vi "Analysis_ELV_From_CVS.vi"() -> ()   [LabVIEW 2018]
uses:
  <vilib>/Utility/file.llb/Read Delimited Spreadsheet (DBL).vi
  <vilib>/imath/engines/lvmath2/RunTimeEngine/RangeToken/NIMS_Range.vi
  <instcachedir>/0/NIMS_Range_846134F467D14A349F7C6CCEF459CDB2.lvgen/NIMS_Range_846134F467D14A349F7C6CCEF459CDB2_000.vi
  <vilib>/imathl/engines/lvmath/Functions/Error Handling/Create Error.vi
  <vilib>/imath/engines/lvmath2/RunTimeEngine/BuiltInFunctions/length/NIMS_length(GV).vi
  <instcachedir>/0/NIMS_length(GV)_08A3D13377FD4E4B96F5795FBF3698FA.lvgen/NIMS_length(GV)_08A3D13377FD4E4B96F5795FBF3698FA_000.vi
  <vilib>/imath/engines/lvmath2/RunTimeEngine/RangeToken/NIMS_Range_R2 - Integer.vi
  <instcachedir>/0/NIMS_Range_R2 - Integer_E35B921DECF84AADB7325A02D418BFCC.lvgen/NIMS_Range_R2 - Integer_E35B921DECF84AADB7325A02D418BFCC_000.vi
  <vilib>/imath/engines/lvmath2/RunTimeEngine/CommandStatement/MC_CommandStatement_break.vi
  <vilib>/imath/engines/lvmath2/RunTimeEngine/IndexRead/NIMS V(S).vi
  <instcachedir>/0/NIMS V(S)_0488751826AF41519A22953C041130DC.lvgen/NIMS V(S)_0488751826AF41519A22953C041130DC_000.vi
  <vilib>/imath/engines/lvmath2/RunTimeEngine/BuiltInFunctions/rem/NIMS_rem_no checks.vi
  <instcachedir>/0/NIMS_rem_no checks_268F985FDA964107BCCF66D5C0ADFD07.lvgen/NIMS_rem_no checks_268F985FDA964107BCCF66D5C0ADFD07_000.vi
  <vilib>/imath/engines/lvmath2/RunTimeEngine/VariableToken/NIMS_VariableToken_CondDefinedDefinedByReplace.vi
  <instcachedir>/0/NIMS_VariableToken_CondDefinedDefinedByReplace_D162CFFC24174562A9FEA619A91E1A56.lvgen/NIMS_VariableToken_CondDefinedDefinedByReplace_D162CFFC24174562A9FEA619A91E1A56_002.vi
  <vilib>/imath/engines/lvmath2/RunTimeEngine/IndexReplace/NIMS V(S)=S.vi
  <instcachedir>/0/NIMS V(S)=S_420DA4522869420292A92FA3CC108C4E.lvgen/NIMS V(S)=S_420DA4522869420292A92FA3CC108C4E_000.vi
  <vilib>/imath/engines/lvmath2/RunTimeEngine/VariableToken/NIMS_VariableToken_CondDefined.vi
  <instcachedir>/0/NIMS_VariableToken_CondDefined_BADDB804EBCA4B86883699DABD34B224.lvgen/NIMS_VariableToken_CondDefined_BADDB804EBCA4B86883699DABD34B224_003.vi
  <vilib>/imath/engines/lvmath2/RunTimeEngine/BuiltInFunctions/interpolate1d/NIMS_interpolate1d(RV,RV,RV,Str).vi
  <vilib>/imath/engines/lvmath2/RunTimeEngine/ErrorHandling/NIMS_Create Error From Enums.vi
  <vilib>/imath/engines/lvmath/Functions/Error Handling/MergeErrorsWrapper.vi
  <vilib>/imath/engines/lvmath2/RunTimeEngine/NodeEndStatement/NIMS_NodeEndStatement_Output.vi
  <instcachedir>/0/NIMS_NodeEndStatement_Output_53EC0D466D134D7ABD903AC30B43404B.lvgen/NIMS_NodeEndStatement_Output_53EC0D466D134D7ABD903AC30B43404B_001.vi
  <instcachedir>/0/NIMS_NodeEndStatement_Output_53EC0D466D134D7ABD903AC30B43404B.lvgen/NIMS_NodeEndStatement_Output_53EC0D466D134D7ABD903AC30B43404B_005.vi
  <vilib>/imath/engines/lvmath2/RunTimeEngine/ErrorHandling/NIMS_Finalize Error.vi
panel:
  out "out2":dbl=0.071713257355
  out "out1":dbl=0.0297284806645
  in  "Tab Control":T1(tab)=enum."Confirming tn equation by comparing curves"
  out "Before Normalization":cluster{"all rows":dbl[], "all rows":dbl[]}(graph)
  out "After Normalization":cluster{"all rows":dbl[], "all rows":dbl[]}(graph)
  out "Emax":dbl=3.25
  out "tmax":dbl=0.2957
  out "E0":dbl=0.006655 format="%_10g"
  in  "Ed":dbl=0.006655
  in  "b":dbl=0.3
  in  "a":dbl=0.16
  in  "Num Cycles":dbl=5.0
  in  "HR":dbl=90.0
  in  "dt":dbl=0.0001
  in  "t0":dbl
  out "XY Graph":cluster{"tnvec":dbl[], "Ev":dbl[]}[](graph)
  out "min value":dbl
  in  "After normalization":path=path "C:/Users/suraj/Documents/Academic/Thesis - Physiological Control/From Ethan/Model1_EKF_12stateCVS/From_CVS_ELV_Norm.txt"
  in  "Original from Jeff":path=path "C:/Users/suraj/Documents/Academic/Thesis - Physiological Control/From Ethan/Model1_EKF_12stateCVS/From_CVS_Elv.txt"
  # "HR was set to 60 bpm"
  # "ts = a + b*tc"
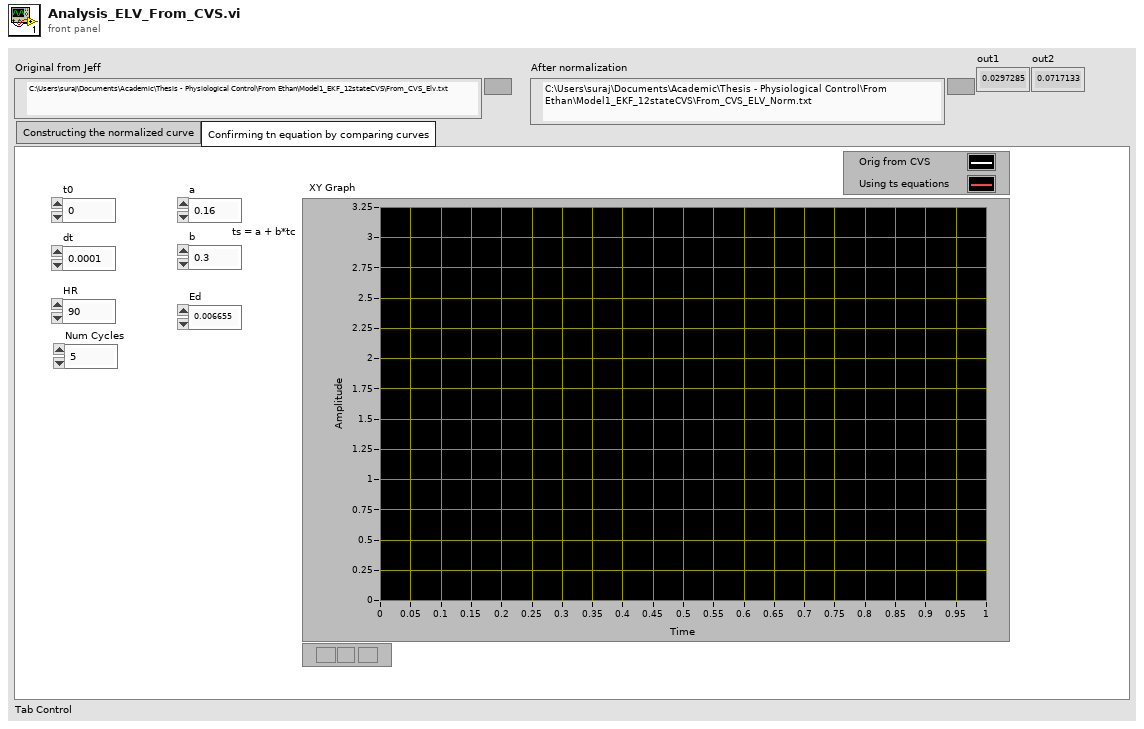
[diagram p1: front panel]
types:
  T1 = enum32{"Constructing the normalized curve", "Confirming tn equation by comparing curves"}
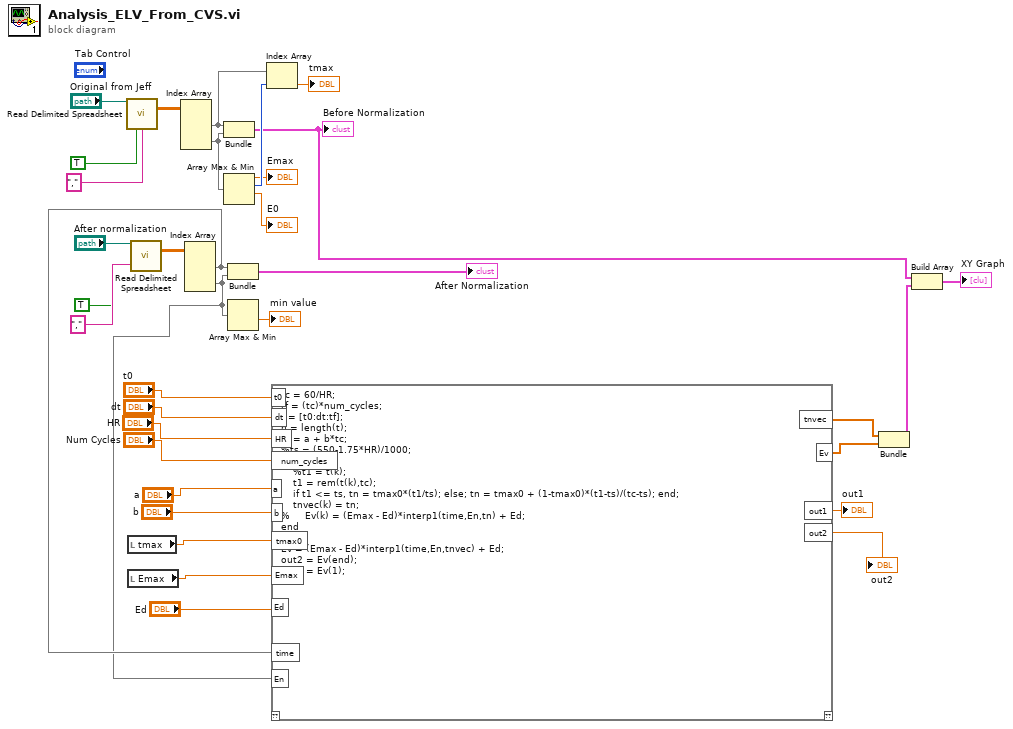
[diagram p0: block diagram]
diagram:
  n1 = call-poly <vilib>:"Read Delimited Spreadsheet.vi"("file path (dialog if empty)"="Original from Jeff", "transpose? (F)"=TRUE, "delimiter (\\t)"="," ("delimiter (\\t)")) -> ("all rows"=w31:dbl[][])  [unwired: 7 in, 5 out]
  n2 = local read "tmax"() -> (w13:dbl)
  n3 = local read "Emax"() -> (w12:dbl)
  n4 = call-poly <vilib>:"Read Delimited Spreadsheet.vi"("file path (dialog if empty)"="After normalization", "transpose? (F)"=TRUE, "delimiter (\\t)"="," ("delimiter (\\t)")) -> ("all rows"=w25:dbl[][])  [unwired: 7 in, 5 out]
  n5 = Index Array(array=w31) -> (element #1=w20:dbl[], element #2=w23:dbl[])  [unwired: 4 in]
  n6 = Index Array(array=w25) -> (element #1=w10:dbl[], element #2=w9:dbl[])  [unwired: 4 in]
  n7 = Bundle("all rows"=w20, "all rows"=w23) -> (w3:cluster{"all rows":dbl[], "all rows":dbl[]})  [unwired: 1 in]
  "Before Normalization" <- w3
  n8 = Array Max & Min(array=w23) -> (max value=→"Emax":dbl, max index (indices)=w30:i32, min value=→"E0":dbl)  [unwired: 1 out]
  n9 = Bundle("all rows"=w10, "all rows"=w9) -> (→"After Normalization":cluster{"all rows":dbl[], "all rows":dbl[]})  [unwired: 1 in]
  n10 = Array Max & Min(array=w9) -> (min value=→"min value":dbl)  [unwired: 3 out]
  n11 = Index Array(array=w20, index=w30) -> (element=→"tmax":dbl)
  n12 = mathscript code="tc = 60/HR;\ntf = (tc)*num_cycles;\nt = [t0:dt:tf];\nn = length(t);\nts = a + b*tc;\n%ts = (550-1.75*HR)/1000;\nfor k = 1:n\n    %t1 = t(k);\n    t1 = rem(t(k),tc);\n    if t1 <= ts, tn = tmax0*(t1/ts); else; tn = tmax0 + (1-tmax0)*(t1-ts)/(tc-ts); end;\n    tnvec(k) = tn;\n%     Ev(k) = (Emax - Ed)*interp1(time,En,tn) + Ed;\nend\n\nEv = (Emax - Ed)*interp1(time,En,tnvec) + Ed;\nout2 = Ev(end);\nout1 = Ev(1);"("t0"="t0", "dt"="dt", "HR"="HR", "num_cycles"="Num Cycles", "a"="a", "b"="b", "tmax0"=w13, "Emax"=w12, "Ed"="Ed", "time"=w10, "En"=w9) -> ("Ev"=w8:dbl[], "tnvec"=w7:dbl[], "out1"=→"out1":dbl, "out2"=→"out2":dbl)  [unwired: 1 in, 1 out]
  n13 = Bundle("tnvec"=w7, "Ev"=w8) -> (w5:cluster{"tnvec":dbl[], "Ev":dbl[]})  [unwired: 1 in]
  n14 = Build Array(w3, w5) -> (→"XY Graph":cluster{"tnvec":dbl[], "Ev":dbl[]}[])
